vi "MouseZoomX.vi"(9 "XY":cluster{"X":dbl, "Y":dbl}, 10 "Delta":i32, 11 "XYGraph输入":refnum<vi>) -> ()   [LabVIEW 2015]
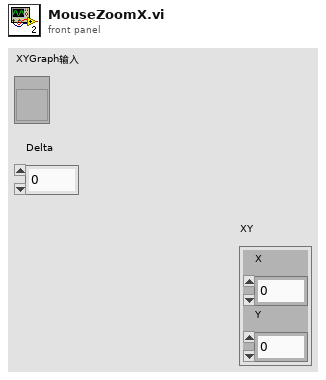
[diagram p1: front panel]
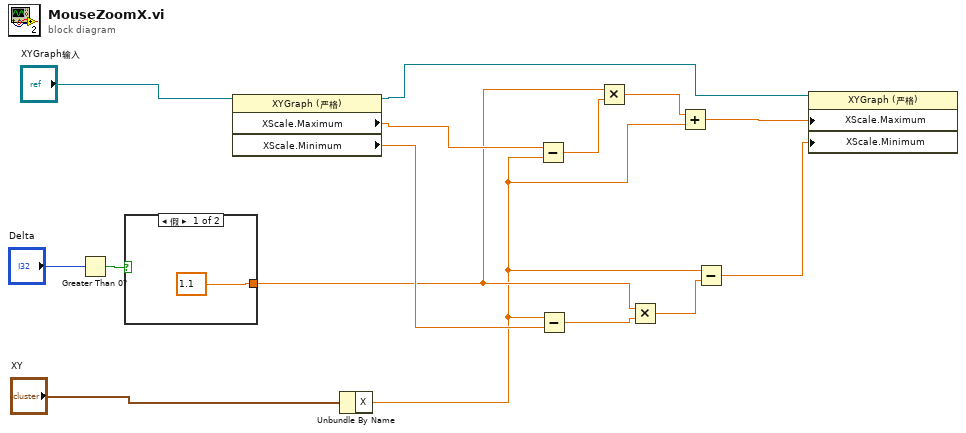
[diagram p0: block diagram]
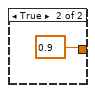
[diagram p2: hidden frame]
diagram:
  n1 = Greater Than 0?(x="Delta") -> (x > 0?=w15:bool)
  n2 = case shown="假" w15 {
    tunnel: [1.1 0.9] -> w5
    frame False {
    }
    frame True {
    }
  }
  n3 = property class="XYGraph (严格)"(reference="XYGraph输入") -> (reference out=w1:refnum<vi>, "XScale.Maximum"=w11:dbl, "XScale.Minimum"=w7:dbl)  [unwired: 1 in, 1 out]
  n4 = Unbundle By Name("XY") -> ("X"=w4:dbl)
  n5 = Subtract(x=w11, y=w4) -> (x-y=w10:dbl)
  n6 = Subtract(x=w4, y=w7) -> (x-y=w6:dbl)
  n7 = Multiply(x=w5, y=w10) -> (x*y=w9:dbl)
  n8 = Multiply(x=w5, y=w6) -> (x*y=w3:dbl)
  n9 = Add(x=w9, y=w4) -> (x+y=w8:dbl)
  n10 = Subtract(x=w4, y=w3) -> (x-y=w2:dbl)
  n11 = property class="XYGraph (严格)"(reference=w1, "XScale.Maximum"=w8, "XScale.Minimum"=w2) -> ()  [unwired: 1 in, 2 out]
